vi "Z Aux Direct Singl Move.vi"(8 "error in (no error)":errorcluster caption="错误输入（无错误）", 9 "fdistance":sgl, 10 "iaxis":i32, 11 "handle":u32) -> (0 "error out":errorcluster caption="错误输出", 2 "function return":i32, 3 "handle out":u32)   [LabVIEW 2015, in "zauxdll.lvlib"]
doc: "int32 __stdcall ZAux_Direct_Singl_Move(ZMC_HANDLE handle, int iaxis, float fdistance);"
uses:
  zauxdll.lvlib
  zauxdll.dll
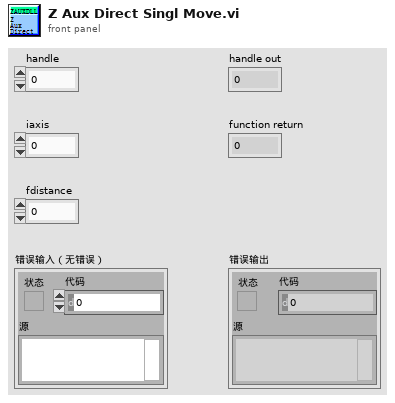
[diagram p1: front panel]
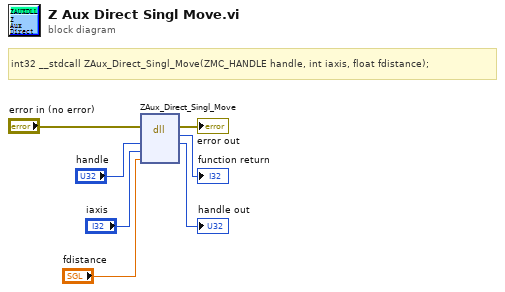
[diagram p0: block diagram]
diagram:
  # "int32 __stdcall ZAux_Direct_Singl_Move(ZMC_HANDLE handle, int iaxis, float fdistance);"
  n1 = dll-call lib="D:/vicomm case/cub/0717/15/Main Folder/Radar - 2015 32bit_autoqueue_angle_0319/zauxdll-2014/zauxdll.*" fn="ZAux_Direct_Singl_Move"(error in="error in (no error)", "handle"="handle", "iaxis"="iaxis", "fdistance"="fdistance") -> (error out=→"error out":errorcluster, →"function return":i32, "handle"=→"handle out":u32)  [unwired: 4 in, 1 out]
